vi "Error Encoder.vi"(4 "error in (no error)":errorcluster) -> (0 "error out":errorcluster)   [LabVIEW 2015, in "StdOut Operations.lvlib"]
uses:
  StdOut Operations.lvlib
  _subVIs/Append String to StdOut.vi
  Data Manipulation/Data Manipulation.lvlib
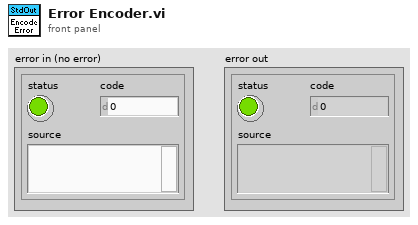
[diagram p1: front panel]
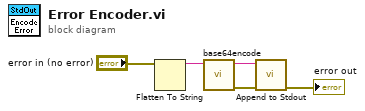
[diagram p0: block diagram]
diagram:
  n1 = Flatten To String(anything="error in (no error)") -> (data string=w1:string)  [unwired: 3 in, 2 out]
  n2 = call "base64encode.vi"("string in (not encoded)"=w1) -> ("Error Out"=w2:errorcluster, "string out (base64-encoded)"=w3:string)  [unwired: 5 in]
  n3 = call-poly "Append to Stdout.vi"("error in (no error)"=w2, "text"=w3) -> ("error out"=→"error out":errorcluster)  [unwired: 5 in]
